vi "SendToReceiver.vi"(8 "error in (no error)":errorcluster, 11 "Communication in":refnum<class "Communication.lvclass">) -> (0 "error out":errorcluster, 3 "Communication out":refnum<class "Communication.lvclass">)   [LabVIEW 2023, in "Communication.lvclass"]
uses:
  Communication.lvclass
  TypeDefs/UserEventOperations.ctl
  TypeDefs/UserEventDataCluster.ctl
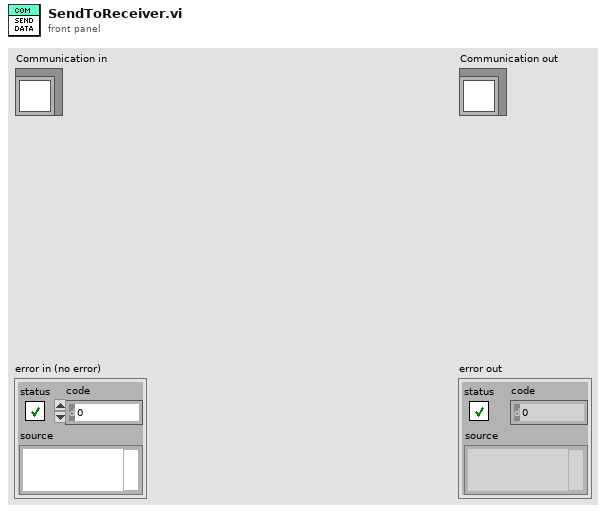
[diagram p1: front panel]
types:
  T1 = typedef "UserEventDataCluster.ctl" = cluster{"State":string, "Data":variant}
  T2 = typedef "UserEventOperations.ctl" = enum16{"Create", "Generate", "Release"}
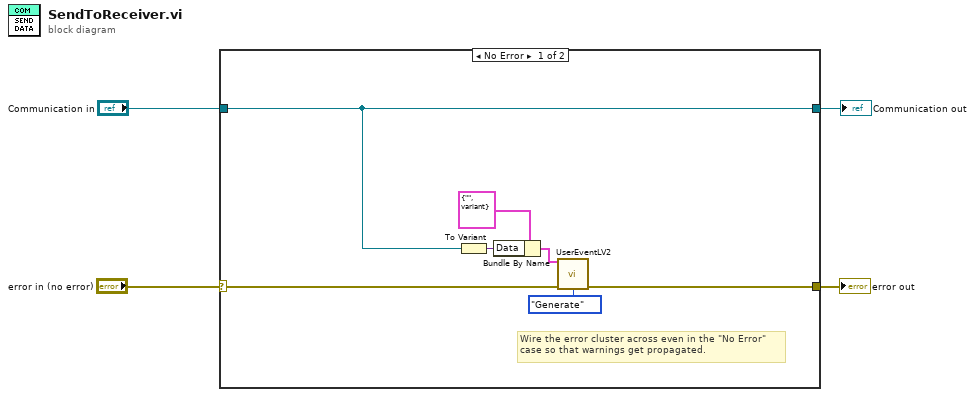
[diagram p0: block diagram]
diagram:
  n1 = case shown="No Error" "error in (no error)" {
    selector: "error in (no error)" -> [w7 w13]
    tunnel: [w6 w13] -> w3
    tunnel: [w5 w12] -> w1
    tunnel: "Communication in" -> [w5 w12]
    frame No Error {
      # "Wire the error cluster across even in the \"No Error\"\ncase so that warnings get propagated."
      n2 = To Variant(anything=w5) -> (Variant=w10:variant)
      n3 = Bundle By Name(cluster=T1 {"State"="", "Data"=variant} ("Data"), "Data"=w10) -> (w8:T1)
      n4 = call "UserEventLV2.vi"("Data"=w8, "Error In"=w7, "Operation"=UserEventOperations."Generate") -> ("Error Out"=w6:errorcluster)  [unwired: 11 in, 1 out]
    }
    frame Error {
    }
  }
  "error out" <- w3
  "Communication out" <- w1
